vi "CH_LM Calibration PyroOffset DAC.vi"(0 "Meter Index":i32, 2 "PYRO DAC Offset (0)":u16, 5 "error in (no error)":errorcluster, 7 "Timeout / ms (3000)":i32=3000, 8 "Action (query)":bool, 9 "Lock Timeout / ms (1000)":i32=1000) -> (11 "Lock timed out":bool, 14 "Meter Index":i32, 16 "PYRO DAC Offset":u16, 19 "error out":errorcluster)   [LabVIEW 2012, in "CH_LM.lvlib"]
doc: "This VI writes a persistent value to the meter that is written to the pyro DAC for calibration of the pyro circuit. The value is stored in the meter and written to the pyro DAC each time the meter powers up."
uses:
  CH_LM.lvlib
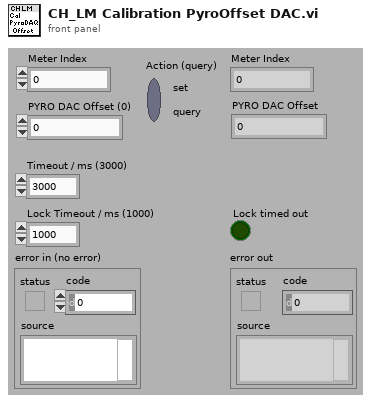
[diagram p1: front panel]
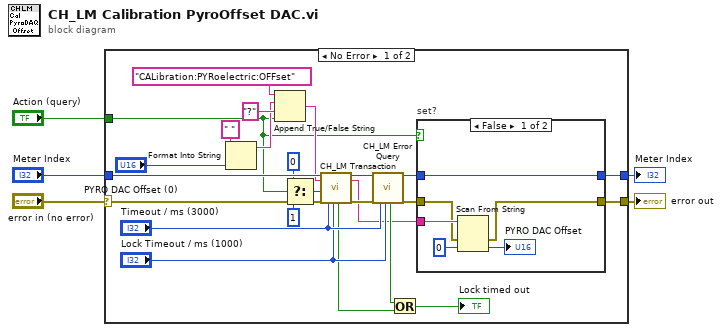
[diagram p0: block diagram]
diagram:
  n1 = case shown="No Error" "error in (no error)" {
    selector: "error in (no error)" -> [w29 w39]
    tunnel: [w9 w39] -> w5
    tunnel: "Meter Index" -> [w28 w38]
    tunnel: [w6 w38] -> w2
    tunnel: "Action (query)" -> [w8 _]
    frame No Error {
      n2 = Format Into String(initial string=" ", "PYRO DAC Offset (0)") -> (resulting string=w17:string)  [unwired: 2 in, 1 out]
      n3 = Append True/False String(1:w8, 2:"?", 3:w17, 4:"CALibration:PYRoelectric:OFFset") -> (0:w16:string)
      n4 = Select(t=0, s=w8, f=1) -> (s? t:f=w15:i32)
      n5 = call "CH_LM Transaction.vi"("Meter Index"=w28, "Command String"=w16, "NofStrings (-1:all)"=w15, "error in (no error)"=w29, "Timeout / ms (3000)"="Timeout / ms (3000)", "Lock Timeout / ms (1000)"="Lock Timeout / ms (1000)") -> ("Lock timed out"=w22:bool, "Meter Index"=w25:i32, "Response"=w11:string, "error out"=w24:errorcluster)  [unwired: 10 out]
      n6 = call "CH_LM Error Query.vi"("Meter Index"=w25, "error in (no error)"=w24, "Timeout / ms (3000)"="Timeout / ms (3000)", "Lock Timeout / ms (1000)"="Lock Timeout / ms (1000)") -> ("Lock timed out"=w23:bool, "Meter Index"=w7:i32, "error out"=w10:errorcluster)  [unwired: 13 out]
      n7 = Or(x=w23, y=w22) -> (x .or. y?=→"Lock timed out":bool)
      n8 = case "set?" shown="False" w8 {
        tunnel: w11 -> [w35 _]
        tunnel: w10 -> [w33 w37]
        tunnel: [w32 w37] -> w9
        tunnel: w7 -> [w30 w36]
        tunnel: [w30 w36] -> w6
        frame False {
          n9 = Scan From String(input string=w35, error in=w33, default 1=u16 0 ("default value 1")) -> (error out=w32:errorcluster, output 1=→"PYRO DAC Offset":u16)  [unwired: 2 in, 2 out]
        }
        frame True {
        }
      }
    }
    frame Error {
    }
  }
  "error out" <- w5
  "Meter Index" <- w2
